vi "is a.vi"(8 "error in (no error)":errorcluster, 11 "Scope in":refnum<class "Scope.lvclass">) -> (0 "error out":errorcluster, 2 "is a":string, 3 "Scope out":refnum<class "Scope.lvclass">)   [LabVIEW 2026, in "Hardware.lvlib" / "Scope.lvclass"]
uses:
  Scope.lvclass
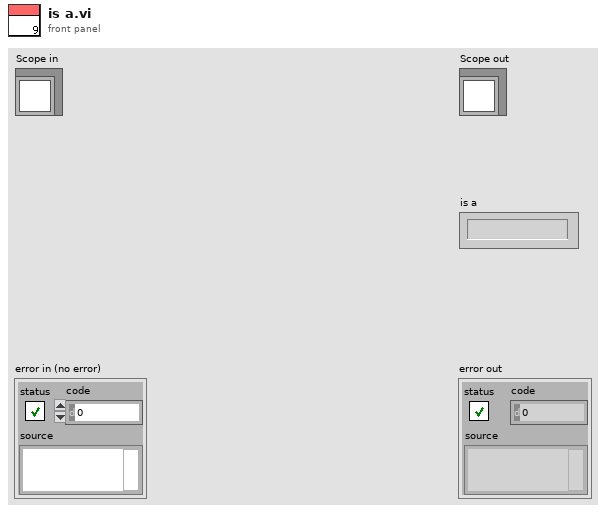
[diagram p1: front panel]
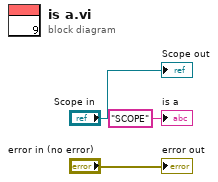
[diagram p0: block diagram]
diagram:
  "error out" <- "error in (no error)"
  "Scope out" <- "Scope in"
  "is a" <- "SCOPE" ("is a")
